vi "Z_OnSw_BtnDown.vi"(8 "error in (no error)":errorcluster, 11 "Z_HSw_in":refnum<class "Z_OnSw.lvclass">) -> (0 "error out":errorcluster, 3 "Z_HSw_out":refnum<class "Z_OnSw.lvclass">)   [LabVIEW 2019, in "Z_OnSw.lvclass"]
uses:
  Z_OnSw.lvclass
  Z_OnSw.lvclass/Z_OnSw.ctl
  switch_state.ctl
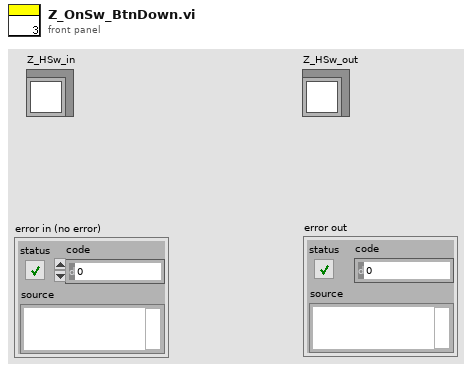
[diagram p1: front panel]
types:
  T1 = typedef "switch_state.ctl" = enum16{"init", "switch off", "not off", "off", "switch on", "not on", "on"}
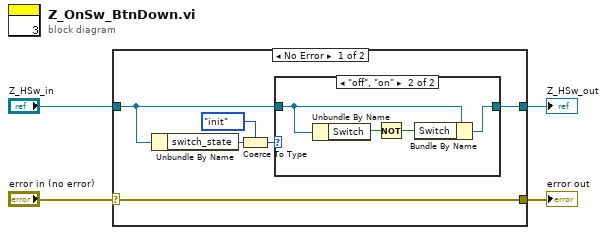
[diagram p0: block diagram]
diagram:
  n1 = case shown="No Error" "error in (no error)" {
    selector: "error in (no error)" -> [w8 w17]
    tunnel: "Z_HSw_in" -> [w6 w16]
    tunnel: [w8 w17] -> w2
    tunnel: [w5 w16] -> w1
    frame No Error {
      n2 = Unbundle By Name(w6) -> ("switch_state"=w10:T1)
      n3 = Coerce To Type(0:w10, 1:switch_state."init" ("switch_state")) -> (2:w7:T1)
      n4 = case shown="\"off\", \"on\"" w7 {
        tunnel: w6 -> [w11 w13]
        tunnel: [w11 w12] -> w5
        frame "init", Default {
        }
        frame "off", "on" {
          n5 = Unbundle By Name(w13) -> ("Switch"=w15:bool)
          n6 = Not(x=w15) -> (.not. x?=w14:bool)
          n7 = Bundle By Name(cluster=w13, "Switch"=w14) -> (w12:refnum<class "Z_OnSw.lvclass">)
        }
      }
    }
    frame Error {
    }
  }
  "Z_HSw_out" <- w1
  "error out" <- w2
